vi "write_attributes.vi"(8 "error in (no error)":errorcluster, 10 "attributes":T1, 11 "NuSVC in":refnum<class "NuSVC.lvclass">) -> (0 "error out":errorcluster, 3 "NuSVC out":refnum<class "NuSVC.lvclass">)   [LabVIEW 2020, in "NuSVC.lvclass"]
uses:
  NuSVC.lvclass
  Controls/nu_svc_attributes.ctl
  NuSVC.lvclass/NuSVC.ctl
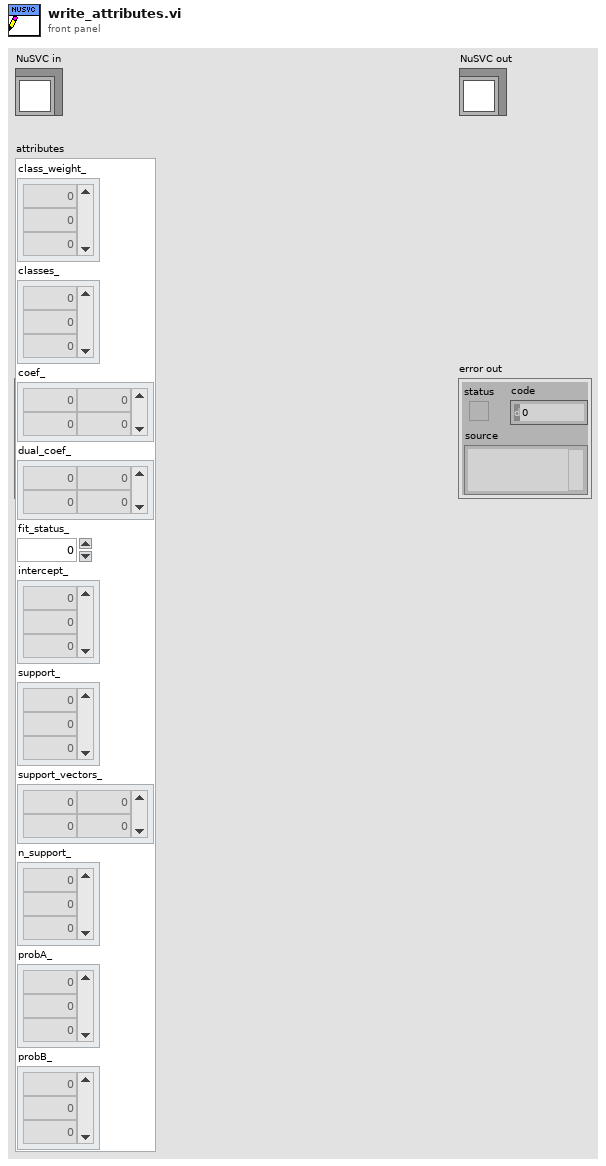
[diagram p1: front panel]
types:
  T1 = typedef "nu_svc_attributes.ctl" = cluster{"class_weight_":dbl[], "classes_":dbl[], "coef_":dbl[][], "dual_coef_":dbl[][], "fit_status_":dbl, "intercept_":dbl[], "support_":dbl[], "support_vectors_":dbl[][], "n_support_":dbl[], "probA_":dbl[], "probB_":dbl[]}
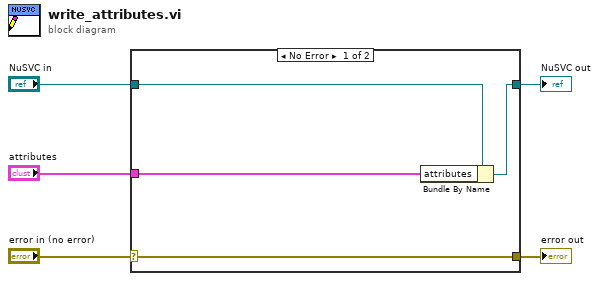
[diagram p0: block diagram]
diagram:
  n1 = case shown="No Error" "error in (no error)" {
    selector: "error in (no error)" -> [w9 w10]
    tunnel: [w9 w10] -> w4
    tunnel: [w7 w11] -> w2
    tunnel: "NuSVC in" -> [w8 w11]
    tunnel: "attributes" -> [w6 _]
    frame No Error {
      n2 = Bundle By Name(cluster=w8, "attributes"=w6) -> (w7:refnum<class "NuSVC.lvclass">)
    }
    frame Error {
    }
  }
  "error out" <- w4
  "NuSVC out" <- w2
